vi "Configure Session.vi"(8 "error in":errorcluster, 11 "Plugin in":refnum<class "Tone Measurements.lvclass">) -> (0 "error out":errorcluster, 3 "Plugin out":refnum<class "Tone Measurements.lvclass">)   [LabVIEW 2025, in "Tone Measurements.lvlib" / "Tone Measurements.lvclass"]
uses:
  Tone Measurements.lvclass
  C:/Program Files/National Instruments/LabVIEW 2025/vi.lib/FlexLogger/SDK/PluginSDK.lvlibp/PEFClasses/SDK/Plugin/Plugin.lvclass
  Tone Measurements.lvclass/Tone Measurements.ctl
  <vilib>/FlexLogger/SDK/PluginSDK.lvlibp/PEFClasses/SDK/Plugin/ParameterAccess/Read DBL.vi
  <vilib>/FlexLogger/SDK/PluginSDK.lvlibp/PEFClasses/SDK/Plugin/ParameterAccess/Read I32.vi
  <vilib>/FlexLogger/SDK/PluginSDK.lvlibp/PEFClasses/SDK/Plugin/Plugin.lvclass
  <vilib>/addons/_NISVFA/_Shared subVIs/Data Objects/Waveforms (DBL)/Waveforms (N Ch).lvclass
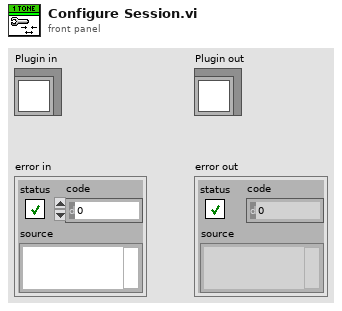
[diagram p1: front panel]
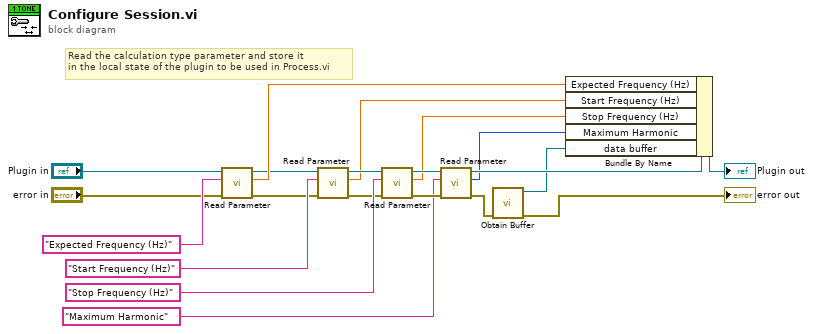
[diagram p0: block diagram]
diagram:
  # "Read the calculation type parameter and store it\nin the local state of the plugin to be used in Process.vi"
  n1 = call-poly <vilib>:"Read Parameter.vi"("error in (no error)"="error in", "Name"="Expected Frequency (Hz)", "Plugin in"="Plugin in") -> ("error out"=w3:errorcluster, "Value"=w16:dbl, "Plugin out"=w11:refnum<class "Tone Measurements.lvclass">)  [unwired: 5 in, 1 out]
  n2 = call-poly <vilib>:"Read Parameter.vi"("Name"="Start Frequency (Hz)", "Plugin in"=w11) -> ("Value"=w6:dbl, "Plugin out"=w12:refnum<class "Tone Measurements.lvclass">)  [unwired: 6 in, 2 out]
  n3 = call-poly <vilib>:"Read Parameter.vi"("Name"="Stop Frequency (Hz)", "Plugin in"=w12) -> ("error out"=w14:errorcluster, "Value"=w5:dbl, "Plugin out"=w13:refnum<class "Tone Measurements.lvclass">)  [unwired: 6 in, 1 out]
  n4 = call-poly <vilib>:"Read Parameter.vi"("error in (no error)"=w14, "Name"="Maximum Harmonic", "Plugin in"=w13) -> ("Value"=w4:i32, "Plugin out"=w10:refnum<class "Tone Measurements.lvclass">)  [unwired: 5 in, 2 out]
  n5 = call <vilib>:"Obtain Buffer.vi"("error in (no error)"=w3) -> ("error out"=→"error out":errorcluster, "buffer out"=w1:refnum<data-value>)  [unwired: 9 in]
  n6 = Bundle By Name(cluster=w10, "Expected Frequency (Hz)"=w16, "Start Frequency (Hz)"=w6, "Stop Frequency (Hz)"=w5, "Maximum Harmonic"=w4, "data buffer"=w1) -> (→"Plugin out":refnum<class "Tone Measurements.lvclass">)
